vi "GetConnectedStatus.vi"(7 "dvr connected":T1) -> (2 "status":T2, 3 "dvr connected":T1)   [LabVIEW 2017, in "ServerComm.lvlib"]
uses:
  <vilib>/addons/InsightCM/Devices/Shared/Common/ServerComm/ServerComm.lvlib
  <vilib>/addons/InsightCM/Devices/Shared/Common/ServerComm/controls/ConnectionStatus.ctl
  <vilib>/addons/InsightCM/Devices/Shared/Common/ServerComm/controls/ConnectedStatusDvr.ctl
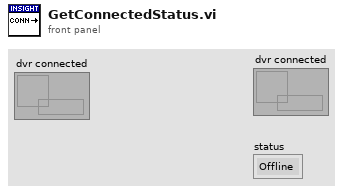
[diagram p1: front panel]
types:
  T1 = typedef "ServerComm.lvlib/ConnectedStatusDvr.ctl" = refnum<data-value>
  T2 = typedef "ServerComm.lvlib/ConnectionStatus.ctl" = enum16{"Offline", "NotAuthorized", "Online"}
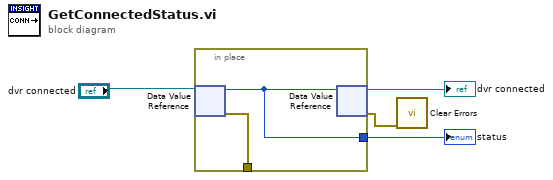
[diagram p0: block diagram]
diagram:
  n1 = in-place {
    in-place-border: [w6] -> w1
    in-place-border: [w5] -> _
    n2 = in-place-dvr #1("dvr connected") -> (w6:T2, w5:errorcluster)
    n3 = in-place-dvr #1(w6) -> (→"dvr connected":T1, w4:errorcluster)
  }
  "status" <- w1
  n4 = call <vilib>:"Clear Errors.vi"("error in (no error)"=w4) -> ()  [unwired: 5 in, 2 out]
